vi "ProgressWindow.vi"(0 "ClassWriter in":refnum<class "ClassWriter.lvclass">, 1 "Message(Exit)":string="Exit", 5 "error in (no error)":errorcluster) -> (14 "ClassWriter out":refnum<class "ClassWriter.lvclass">, 19 "error out":errorcluster)   [LabVIEW 2016, in "ClassWriter.lvclass"]
uses:
  <resource>/Framework/Providers/Open_GDS/ClassProviders/Provider_BaseClassInterface/ClassWriter_class/ClassWriter.lvclass
  <resource>/Framework/Providers/Open_GDS/ClassProviders/Provider_BaseClassInterface/ClassWriter_class/ClassWriter.lvclass/ClassWriter.ctl
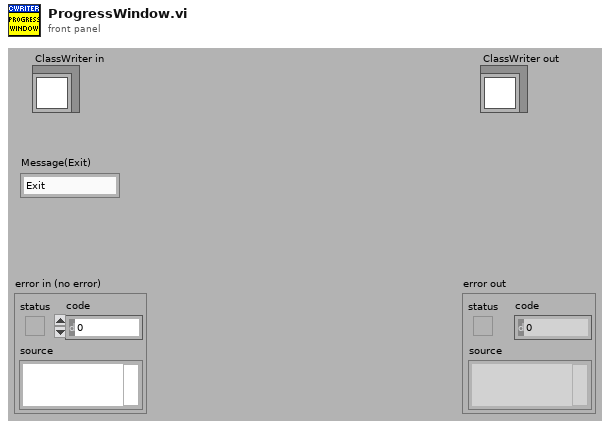
[diagram p1: front panel]
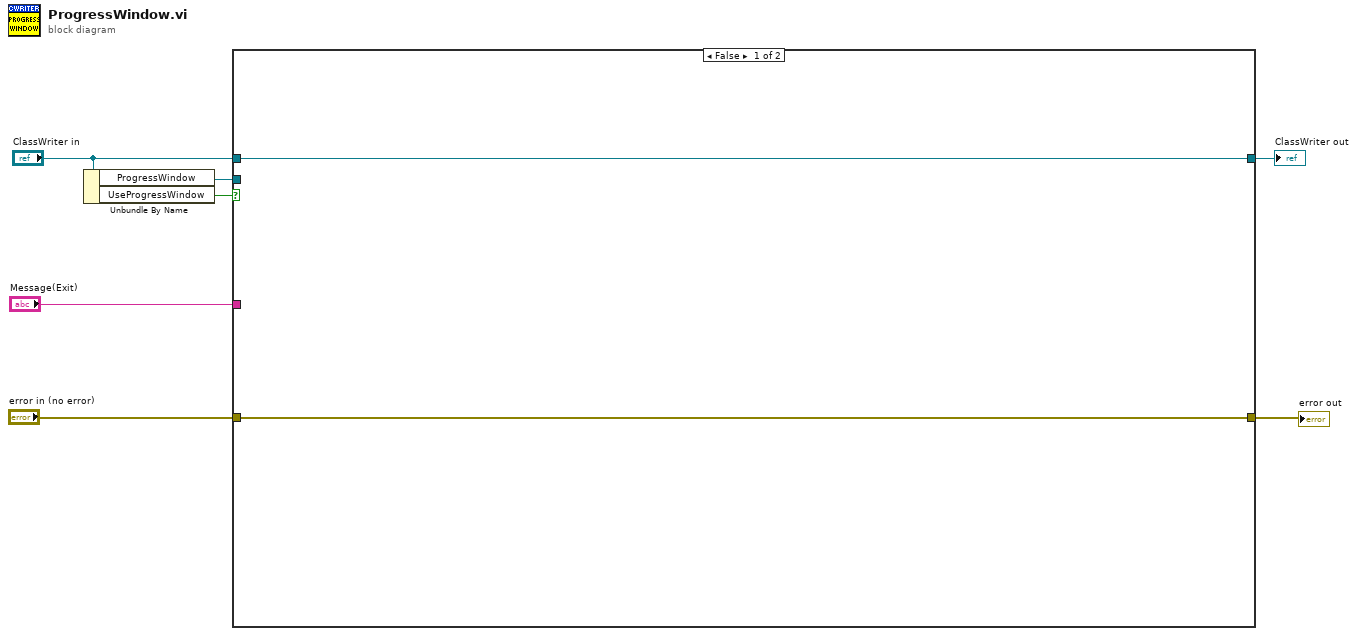
[diagram p0: block diagram]
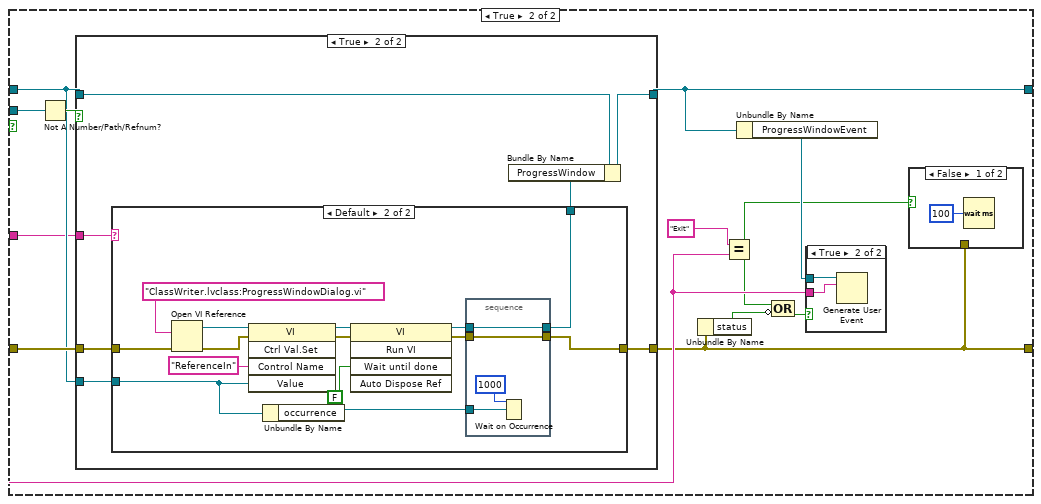
[diagram p2: hidden frame]
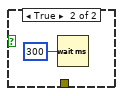
[diagram p4: hidden frame]
diagram:
  n1 = Unbundle By Name("ClassWriter in") -> ("ProgressWindow"=w7:refnum<vi>, "UseProgressWindow"=w1:bool)
  n2 = case shown="False" w1 {
    tunnel: w7 -> [_ w21]
    tunnel: "error in (no error)" -> [w9 w19]
    tunnel: [w8 w18] -> w5
    tunnel: "ClassWriter in" -> [w8 w16]
    tunnel: "Message(Exit)" -> [_ w15]
    tunnel: [w9 w13] -> w2
    frame False {
    }
    frame True {
      n3 = Not A Number/Path/Refnum?(number/path/refnum=w21) -> (NaN/Path/Refnum?=w20:bool)
      n4 = case shown="True" w20 {
        tunnel: w19 -> [w26 w34]
        tunnel: w16 -> [_ w33]
        tunnel: w16 -> [w27 w32]
        tunnel: [w27 w31] -> w18
        tunnel: [w26 w29] -> w13
        tunnel: w15 -> [_ w28]
        frame False {
        }
        frame True {
          n5 = case shown="Default" w28 {
            tunnel: w34 -> [w35 w49]
            tunnel: w33 -> [_ w42]
            tunnel: [_ w38] -> w30
            tunnel: [w35 w37] -> w29
            frame "Exit", "Hide", "UnHide" {
            }
            frame Default {
              n6 = Open VI Reference(vi path="ClassWriter.lvclass:ProgressWindowDialog.vi", error in (no error)=w49) -> (vi reference=w47:refnum<vi>, error out=w46:errorcluster)  [unwired: 4 in]
              n7 = invoke class="VI" method="Ctrl Val.Set"(reference=w47, error in=w46, "Control Name"="ReferenceIn", "Value"=w42) -> (reference out=w44:refnum<vi>, error out=w43:errorcluster)  [unwired: 1 in, 3 out]
              n8 = Unbundle By Name(w42) -> ("occurrence"=w41:refnum<k4>)
              n9 = invoke class="VI" method="Run VI"(reference=w44, error in=w43, "Wait until done"=FALSE ("Wait Until Done")) -> (reference out=w40:refnum<vi>, error out=w39:errorcluster)  [unwired: 2 in, 3 out]
              n10 = stacked-sequence {
                tunnel: w41 -> [w51]
                tunnel: w40 -> [w53]
                tunnel: w39 -> [w52]
                tunnel: [w53] -> w38
                tunnel: [w52] -> w37
                frame #0 {
                  n11 = Wait on Occurrence(2:w51, 3:1000 ("ms timeout (-1)")) -> ()  [unwired: 1 in, 1 out]
                }
              }
            }
          }
          n12 = Bundle By Name(cluster=w32, "ProgressWindow"=w30) -> (w31:refnum<class "ClassWriter.lvclass">)
        }
      }
      n13 = Unbundle By Name(w13) -> ("status"=w12:bool)
      n14 = Equal?(x="Exit", y=w15) -> (x = y?=w10:bool)
      n15 = Unbundle By Name(w18) -> ("ProgressWindowEvent"=w17:refnum<user-event>)
      n16 = Compound Arithmetic op=OR(w10, invert w12) -> (w11:bool)
      n17 = case shown="True" w11 {
        tunnel: w17 -> [_ w23]
        tunnel: w15 -> [_ w22]
        frame False {
        }
        frame True {
          n18 = Generate User Event(user event=w23, event data cluster=w22) -> ()  [unwired: 2 in, 2 out]
        }
      }
      n19 = case shown="False" w10 {
        tunnel: w13 -> [_ _]
        frame False {
          n20 = Wait (ms)(milliseconds to wait=u32 100) -> ()  [unwired: 1 out]
        }
        frame True {
          n21 = Wait (ms)(milliseconds to wait=u32 300) -> ()  [unwired: 1 out]
        }
      }
    }
  }
  "error out" <- w2
  "ClassWriter out" <- w5
